vi "Configure Variable Constant.vi"(0 "VISA resource name":refnum<visa-resource-name>, 5 "Variable Const No. (1)":i32=1 min=1 max=100, 9 "Value":dbl=1.0 format="%#_8g", 11 "error in (no error)":errorcluster) -> (4 "VISA resource name out":refnum<visa-resource-name>, 8 "Variable Const No.":i32, 15 "error out":errorcluster)   [LabVIEW 2020, in "Yokogawa GX Series.lvlib"]
doc: "Sets Variable Constants.\n\nCommand: SWConst."
uses:
  <instrlib>/Yokogawa GX Series/Yokogawa GX Series.lvlib
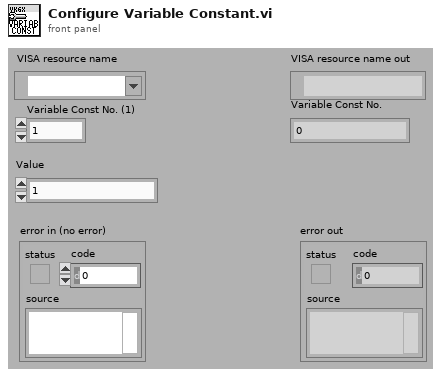
[diagram p1: front panel]
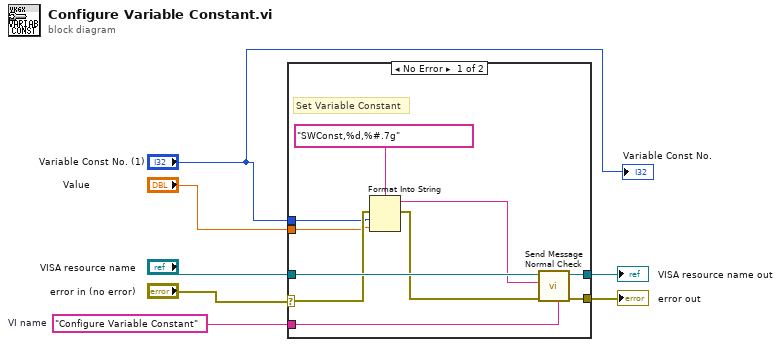
[diagram p0: block diagram]
diagram:
  w3 = "Configure Variable Constant"  # VI name
  n1 = case shown="No Error" "error in (no error)" {
    selector: "error in (no error)" -> [w12 w18]
    tunnel: [w17 w19] -> w7
    tunnel: [w16 w18] -> w6
    tunnel: "VISA resource name" -> [w15 w19]
    tunnel: w3 -> [w11 _]
    tunnel: "Value" -> [w10 _]
    tunnel: "Variable Const No. (1)" -> [w8 _]
    frame No Error {
      # "Set Variable Constant"
      n2 = Format Into String(format string="SWConst,%d,%#.7g", error in=w12, w8, w10) -> (resulting string=w9:string, error out=w13:errorcluster)  [unwired: 1 in]
      n3 = call <instrlib>:"Send Message Normal Check.vi"("Source (\"\")"=w11, "error in (no error)"=w13, "Send Message (\"\")"=w9, "VISA resource name"=w15) -> ("error out"=w16:errorcluster, "VISA resource name out"=w17:refnum<visa-resource-name>)  [unwired: 2 in, 4 out]
    }
    frame Error {
    }
  }
  "error out" <- w6
  "VISA resource name out" <- w7
  "Variable Const No." <- "Variable Const No. (1)"
